vi "concatenate slow zstack raw files.vi"(10 "preset type":string, 11 "slow z root folder":path) -> ()   [LabVIEW 2012]
doc: "SciScan 1.2 160622"
uses:
  MacroGUI Module/SubVIs/Preset VIs/Z-Scan Types.ctl
  GFG/GFGnumericGet.vi
  GFG/GFGpathGet.vi
  GFG/GFG library.lvlib
panel:
  in  "stop":bool
  out "Horizontal Graduated Bar":dbl(slide) caption="Deleting temp files" scale=0.0..4.0
  out "All Files in Dir":path[](array[path])
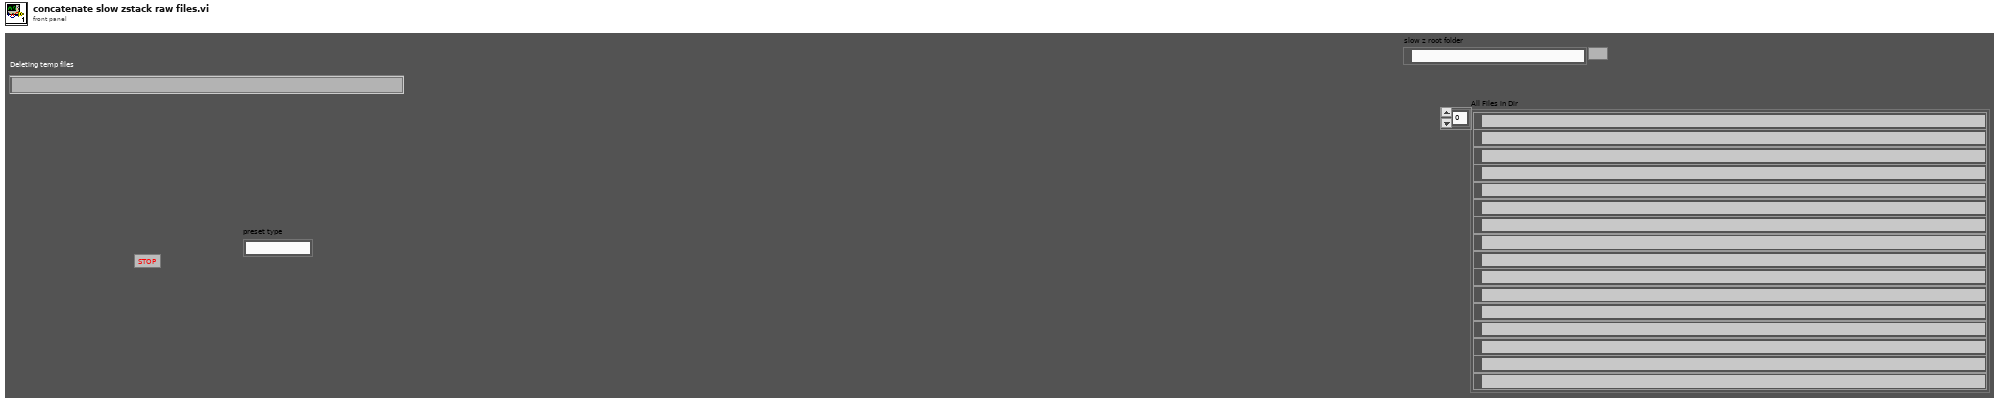
[diagram p1: front panel]
types:
  T1 = enum16{"open", "replace", "create", "open or create", "replace or create", "replace or create with confirmation"}
  T2 = typedef "Z-Scan Types.ctl" = enum16{"Single Plane", "Slow Z", "Z-Stack (Regular)", "Fast Z (Piezo)"}
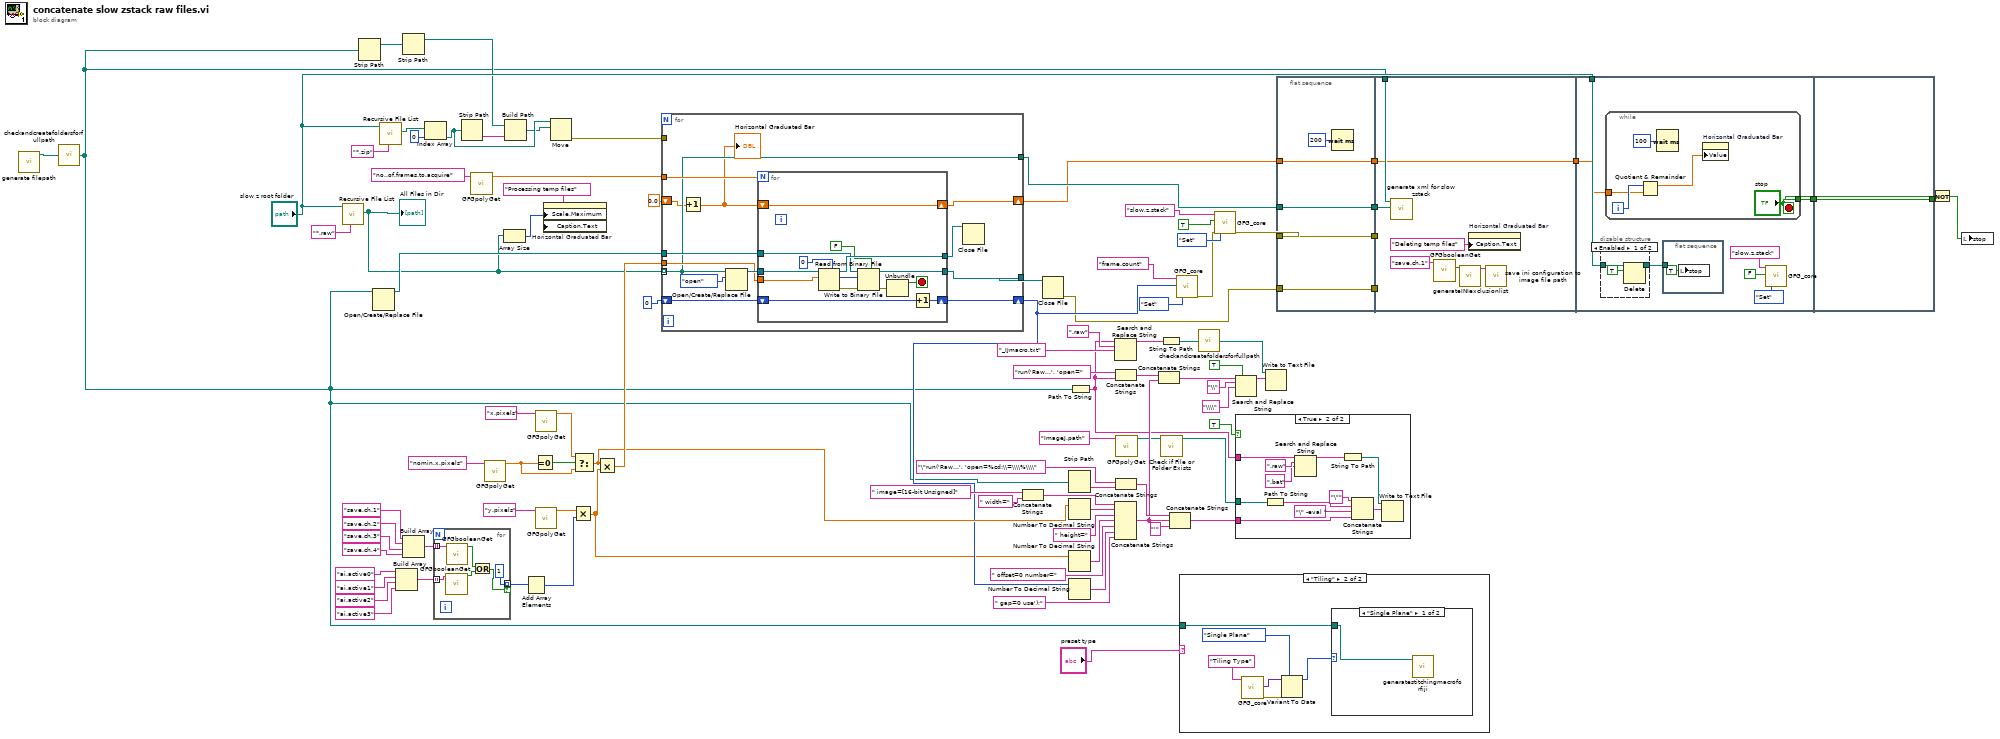
[diagram p0: block diagram]
diagram:
  n1 = call "generate filepath.vi"() -> ("path"=w38:path)  [unwired: 11 in]
  n2 = call "checkandcreatefoldersforfullpath.vi"("Path IN"=w38) -> ("Path OUT"=w1:path)  [unwired: 4 in]
  n3 = call <vilib>:"Recursive File List.vi"("pattern"="*.raw", "Folder Path"="slow z root folder") -> ("All Files in Dir"=w26:path[])  [unwired: 5 in, 4 out]
  "All Files in Dir" <- w26
  n4 = Strip Path(path=w1) -> (stripped path=w22:path)  [unwired: 1 out]
  n5 = Open/Create/Replace File(file path (use dialog)=w1) -> (refnum out=w92:refnum<file>)  [unwired: 5 in, 2 out]
  n6 = call <vilib>:"Recursive File List.vi"("pattern"="*.zip", "Folder Path"="slow z root folder") -> ("All Files in Dir"=w20:path[])  [unwired: 5 in, 4 out]
  n7 = Build Array("ai.active0" ("Variable Name in"), "ai.active1" ("Variable Name in"), "ai.active2" ("Variable Name in"), "ai.active3" ("Variable Name in")) -> (w51:string[])
  n8 = Strip Path(path=w22) -> (stripped path=w21:path)  [unwired: 1 out]
  n9 = Build Array("save.ch.1" ("Variable Name in"), "save.ch.2" ("Variable Name in"), "save.ch.3" ("Variable Name in"), "save.ch.4" ("Variable Name in")) -> (w46:string[])
  n10 = Index Array(array=w20, index=0) -> (element=w17:path)
  n11 = for {
    tunnel: w46 -> [w102] mode=indexing
    tunnel: w51 -> [w101] mode=indexing
    tunnel: [1 ("x+1")] -> w52 mode=indexing if=w98
    n12 = call "GFGbooleanGet.vi"("Variable Name in"=w101) -> ("Boolean Value OUT"=w100:bool)  [unwired: 9 in, 1 out]
    n13 = call "GFGbooleanGet.vi"("Variable Name in"=w102) -> ("Boolean Value OUT"=w99:bool)  [unwired: 9 in, 1 out]
    n14 = Or(x=w99, y=w100) -> (x .or. y?=w98:bool)
  }
  n15 = Strip Path(path=w17) -> (name=w18:string)  [unwired: 1 out]
  n16 = call-poly "GFGpolyGet.vi"("Variable Name in"="no..of.frames.to.acquire") -> ("Numeric"=w94:dbl)  [unwired: 8 in, 2 out]
  n17 = call-poly "GFGpolyGet.vi"("Variable Name in"="nomin.x.pixels") -> ("Numeric"=w53:dbl)  [unwired: 8 in, 2 out]
  n18 = Array Size(array=w26) -> (size(s)=w14:i32)
  n19 = Build Path(base path=w21, name or relative path=w18) -> (appended path=w16:path)
  n20 = Add Array Elements(numeric array=w52) -> (sum=w41:i32)
  n21 = Equal To 0?(x=w53) -> (x = 0?=w55:bool)
  n22 = call-poly "GFGpolyGet.vi"("Variable Name in"="x.pixels") -> ("Numeric"=w54:dbl)  [unwired: 8 in, 2 out]
  n23 = call-poly "GFGpolyGet.vi"("Variable Name in"="y.pixels") -> ("Numeric"=w28:dbl)  [unwired: 8 in, 2 out]
  n24 = property on="Horizontal Graduated Bar" class="Slide (strict)"("Scale.Maximum"=w14, "Caption.Text"="Processing temp files" ("Label.Text")) -> ()  [unwired: 2 in, 2 out]
  n25 = Move(source path=w17, 10:w16) -> (error out=w15:errorcluster)  [unwired: 3 in, 2 out]
  n26 = Multiply(x=w28, y=w41) -> (x*y=w27:dbl)
  n27 = Select(t=w54, s=w55, f=w53) -> (s? t:f=w61:dbl)
  n28 = Multiply(x=w61, y=w27) -> (x*y=w93:dbl)
  n29 = for {
    tunnel: w94 -> [w113]
    tunnel: w93 -> [w112]
    tunnel: w26 -> [w106] mode=indexing
    tunnel: w92 -> [w111]
    shift-right: [w109] -> w36
    shift-left: u16 0 ("element") -> [w110]
    tunnel: [w108] -> w39
    tunnel: [w106] -> w30
    shift-right: [w104] -> w13
    shift-left: 0.0 -> [w105]
    tunnel: w15 -> [_]
    n30 = Increment(x=w105) -> (x+1=w103:dbl)
    "Horizontal Graduated Bar" <- w103
    n31 = Open/Create/Replace File(file path (use dialog)=w106, operation (0:open)=T1."open") -> (refnum out=w114:refnum<file>)  [unwired: 4 in, 2 out]
    n32 = for {
      N: w113 -> [_]
      tunnel: w114 -> [w129]
      tunnel: w112 -> [w127]
      tunnel: [w126] -> w107
      tunnel: w111 -> [w124]
      tunnel: [w123] -> w108
      shift-right: [w117] -> w109
      shift-left: w110 -> [w118]
      shift-right: [w116] -> w104
      shift-left: w103 -> [w116]
      stop <- w119 stop-if-true
      n33 = Read from Binary File(5:u16 0 ("element"), 10:w127, 11:w129) -> (0:w122:errorcluster, 2:w120:u16[], 3:w126:refnum<file>)  [unwired: 3 in, 1 out]
      n34 = Write to Binary File(file (use dialog)=w124, data=w120, error in=w122, 5:FALSE ("prepend array or string size? (T)")) -> (refnum out=w123:refnum<file>, error out=w121:errorcluster)  [unwired: 2 in, 1 out]
      n35 = Unbundle(w121) -> ("status"=w119:bool)  [unwired: 2 out]
      n36 = Increment(x=w118) -> (x+1=w117:u16)
    }
    n37 = Close File(refnum=w107) -> ()  [unwired: 1 in, 2 out]
  }
  n38 = Concatenate Strings(" image=[16-bit Unsigned]" ("image type"), " width=" ("string")) -> (w84:string)
  n39 = Close File(refnum=w39) -> (error out=w9:errorcluster)  [unwired: 1 in, 1 out]
  n40 = Strip Path(path=w1) -> (name=w82:string)  [unwired: 1 out]
  n41 = Number To Decimal String(number=w61) -> (decimal integer string=w91:string)  [unwired: 1 in]
  n42 = Number To Decimal String(number=w27) -> (decimal integer string=w89:string)  [unwired: 1 in]
  n43 = Number To Decimal String(number=w36) -> (decimal integer string=w87:string)  [unwired: 1 in]
  n44 = Path To String(path=w1) -> (string=w73:string)
  n45 = Search and Replace String(input string=w73, search string=".raw", replace string="_IJmacro.txt" ("string")) -> (result string=w68:string)  [unwired: 5 in, 3 out]
  n46 = Concatenate Strings(w84, w91, " height=", w89, " offset=0 number=", w87, " gap=0 use');") -> (w76:string)
  n47 = Concatenate Strings("run('Raw...', 'open=", w73) -> (w77:string)
  n48 = Concatenate Strings("\"run('Raw...', 'open=%cd:\\=\\\\%\\\\", w82) -> (w81:string)
  n49 = call-poly "GFGpolyGet.vi"("Variable Name in"="ImageJ.path" ("Tag in")) -> ("Path"=w65:path)  [unwired: 8 in, 2 out]
  n50 = Concatenate Strings(w77, w76) -> (w69:string)
  n51 = String To Path(string=w68) -> (path=w63:path)
  n52 = call <vilib>:"Check if File or Folder Exists.vi"("path"=w65) -> ("dup path"=w64:path)  [unwired: 8 in, 2 out]
  n53 = Concatenate Strings(w81, w76, "'" ("string")) -> (w79:string)
  n54 = call "GFG_core.vi"("Variable Name in"="frame.count", "Variant in"=w36, "Action"=enum16{"Init", "Set", "Get", "Clear"}."Set") -> ("error out"=w32:errorcluster)  [unwired: 10 in, 6 out]
  n55 = case shown="\"Tiling\"" "preset type" {
    tunnel: w1 -> [_ w130]
    frame "False", Default {
    }
    frame "Tiling" {
      n56 = call "GFG_core.vi"("Variable Name in"="Tiling Type") -> ("Variant Out"=w132:variant, "error out"=w134:errorcluster)  [unwired: 12 in, 5 out]
      n57 = Variant To Data(error in=w134, type=Z-Scan_Types."Single Plane" ("Tiling Type"), Variant=w132) -> (data=w131:T2)  [unwired: 1 out]
      n58 = case shown="\"Single Plane\"" w131 {
        tunnel: w130 -> [w136 _]
        frame "Single Plane" {
          n59 = call "generatestitchingmacroforfiji.vi"("file"=w136) -> ()  [unwired: 11 in]
        }
        frame "Z-Stack (Regular)", Default {
        }
      }
    }
  }
  n60 = call "checkandcreatefoldersforfullpath.vi"("Path IN"=w63) -> ("Path OUT"=w62:path)  [unwired: 4 in]
  n61 = call "GFG_core.vi"("Variable Name in"="slow.z.stack", "Variant in"=TRUE ("replace all? (F)"), "error in (no error)"=w32, "Action"=enum16{"Init", "Set", "Get", "Clear"}."Set") -> ("error out"=w29:errorcluster)  [unwired: 9 in, 6 out]
  n62 = Search and Replace String(replace all?=TRUE ("replace all? (F)"), input string=w69, search string="\\", replace string="\\\\" ("replace string (\"\")")) -> (result string=w67:string)  [unwired: 4 in, 3 out]
  n63 = case shown="True" TRUE {
    tunnel: w79 -> [_ w141]
    tunnel: w73 -> [_ w140]
    tunnel: w64 -> [_ w139]
    frame False {
    }
    frame True {
      n64 = Path To String(path=w139) -> (string=w138:string)
      n65 = Search and Replace String(input string=w140, search string=".raw", replace string=".bat" ("string")) -> (result string=w143:string)  [unwired: 5 in, 3 out]
      n66 = String To Path(string=w143) -> (path=w144:path)
      n67 = Concatenate Strings("\"" ("string"), w138, "\" -eval " ("string"), w141) -> (w142:string)
      n68 = Write to Text File(file (use dialog)=w144, text=w142) -> ()  [unwired: 2 in, 3 out]
    }
  }
  n69 = Write to Text File(file (use dialog)=w62, text=w67) -> ()  [unwired: 2 in, 3 out]
  n70 = flat-sequence {
    tunnel: w9 -> [w149]
    tunnel: w13 -> [w150]
    tunnel: w29 -> [w151]
    tunnel: w30 -> [w152]
    tunnel: [w152] -> w8
    tunnel: [w151] -> w7
    tunnel: [w150] -> w6
    tunnel: [w149] -> w5
    tunnel: w1 -> [w156]
    tunnel: [w155] -> w4
    tunnel: w8 -> [w157]
    tunnel: w7 -> [_]
    tunnel: w6 -> [w155]
    tunnel: w5 -> [_]
    tunnel: "slow z root folder" -> [w163]
    tunnel: w4 -> [w160]
    tunnel: [w161] -> w3
    tunnel: [w176] -> w12
    tunnel: w3 -> [w176]
    frame #0 {
      n71 = Wait (ms)(milliseconds to wait=u32 200) -> ()  [unwired: 1 out]
    }
    frame #1 {
      n72 = call "generate xml for slow zstack.vi"("Old File Path"=w157, "New File Path"=w156) -> ()  [unwired: 10 in]
      n73 = call "GFGbooleanGet.vi"("Variable Name in"="save.ch.1") -> ("Found/Replaced"=w158:bool)  [unwired: 9 in, 1 out]
      n74 = call "generateINIexclusionlist.vi"("T for reso, F for galvo"=w158) -> ("Array"=w159:string[])  [unwired: 10 in]
      n75 = property on="Horizontal Graduated Bar" class="Slide (strict)"("Caption.Text"="Deleting temp files") -> ()  [unwired: 2 in, 2 out]
      n76 = call "save ini configuration to image file path.vi"("exclusion regexp array"=w159) -> ()  [unwired: 11 in]
    }
    frame #2 {
      n77 = disable-structure shown="Enabled" {
        disable-tunnel: w163 -> [w175 _]
        disable-tunnel: [w173 _] -> w162
        frame Enabled {
          n78 = Delete(path (use dialog)=w175, entire hierarchy (F)=TRUE) -> (deleted path=w173:path)  [unwired: 3 in, 2 out]
        }
        frame Disabled {
        }
      }
      n79 = while {
        tunnel: ["stop"] -> w161
        tunnel: w160 -> [w170]
        i -> [w171]
        stop <- "stop" stop-if-true
        n80 = Quotient & Remainder(x=w171, y=w170) -> (x-y*floor(x/y)=w169:dbl)  [unwired: 1 out]
        n81 = Wait (ms)(milliseconds to wait=u32 100) -> ()  [unwired: 1 out]
        n82 = property on="Horizontal Graduated Bar" class="Slide (strict)"("Value"=w169) -> ()  [unwired: 2 in, 2 out]
      }
      n83 = flat-sequence {
        tunnel: w162 -> [_]
        frame #0 {
          n84 = local write "stop"(TRUE ("stop")) -> ()
        }
      }
      n85 = call "GFG_core.vi"("Variable Name in"="slow.z.stack", "Variant in"=FALSE ("replace all? (F)"), "Action"=enum16{"Init", "Set", "Get", "Clear"}."Set") -> ()  [unwired: 10 in, 7 out]
    }
    frame #3 {
    }
  }
  n86 = Not(x=w12) -> (.not. x?=w11:bool)
  n87 = local write "stop"(w11) -> ()
